vi "LoadSteinhartHartCoeff.vi"(8 "error in (no error)":errorcluster) -> (0 "error out":errorcluster)   [LabVIEW 2018, in "Acquisition.lvlib"]
uses:
  Acquisition.lvlib
  <vilib>/Utility/xml.llb/Read From XML File(string).vi
  Global Thermistor Coefficient Array.vi
panel:
  out "value":T1
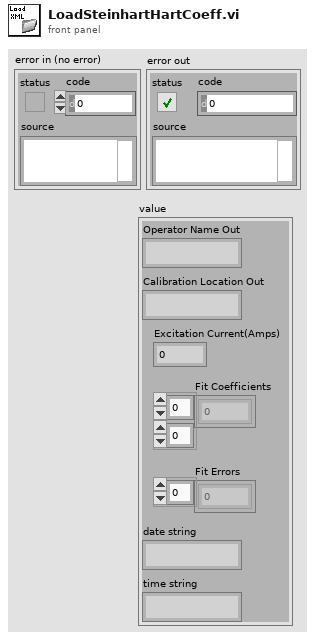
[diagram p1: front panel]
types:
  T1 = cluster{"Operator Name Out":string, "Calibration Location Out":string, "Excitation Current(Amps)":dbl, "Fit Coefficients":dbl[][], "Fit Errors":dbl[], "date string":string, "time string":string}
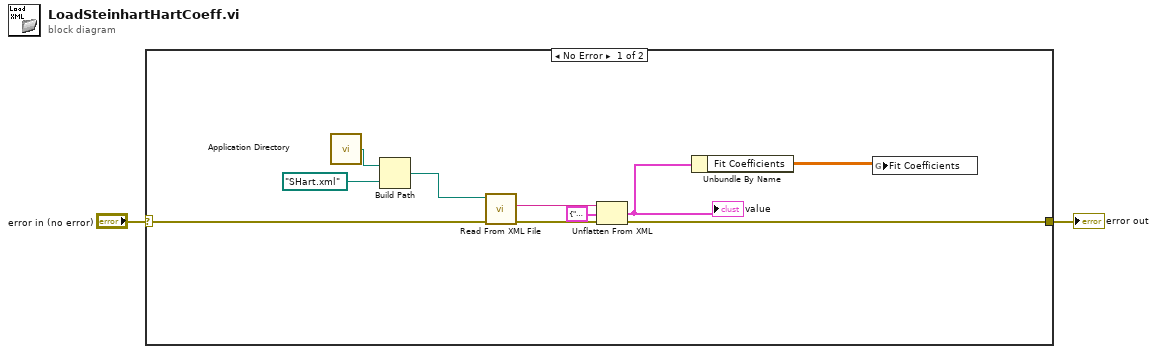
[diagram p0: block diagram]
diagram:
  n1 = case shown="No Error" "error in (no error)" {
    selector: "error in (no error)" -> [w6 w13]
    tunnel: [w7 w13] -> w2
    frame No Error {
      n2 = call <vilib>:"Application Directory.vi"() -> ("Application Directory"=w8:path)
      n3 = Build Path(base path=w8, name or relative path=path "SHart.xml" ("string")) -> (appended path=w11:path)
      n4 = call-poly <vilib>:"Read From XML File.vi"("error in (no error)"=w6, "XML File Path"=w11) -> ("error out"=w9:errorcluster, "XML Elements"=w10:string)  [unwired: 7 in, 1 out]
      n5 = Unflatten From XML(xml string=w10, type=T1 {"Operator Name Out"="", "Calibration Location Out"="", "Excitation Current(Amps)"=0.0, "Fit Coefficients"=[], "Fit Errors"=[], "date string"="", "time string"=""} ("output cluster"), error in (no error)=w9) -> (value=w5:T1, error out=w7:errorcluster)
      "value" <- w5
      n6 = Unbundle By Name(w5) -> ("Fit Coefficients"=w4:dbl[][])
      n7 = global write "Global Thermistor Coefficient Array.vi" "Fit Coefficients"(w4) -> ()
    }
    frame Error {
    }
  }
  "error out" <- w2
